vi "Logging Message Loop.vi"(8 "System Control":refnum<queue>, 10 "Data Queue":refnum<queue>, 11 "Logging":refnum<queue>) -> (0 "error out":errorcluster)   [LabVIEW 2020, in "ChromTech Next Gen Pump.lvlib" / "Logging.lvlib"]
doc: "The message loop subVI to handle messages pertaining to logging data."
uses:
  Logging.lvlib
  support/Message Queue/Message Cluster.ctl
  Instrument Manager/Instrument State.ctl
  Logging State.ctl
  Logging Configuration.ctl
  <vilib>/Utility/error.llb/Error Cluster From Error Code.vi
  <vilib>/Utility/file.llb/Write Delimited Spreadsheet (string).vi
  <vilib>/ErrorRing/Error Ring.xnode
  support/Message Queue/Message Queue.lvlib
  Instrument Manager/Instrument Manager.lvlib
panel:
  in  "error in (no error)":errorcluster
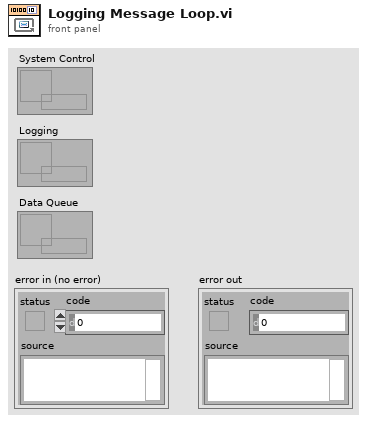
[diagram p1: front panel]
types:
  T1 = typedef "ChromTech Next Gen Pump.lvlib/Logging.lvlib/Logging Configuration.ctl" = cluster{"Log Directory Path":path, "Log File Path":path, "Log File Prefix":string, "Log File Extension":string, "File Delimiter":string, "Header Info":string[][], "Channels":string[], "Log Instrument Runs":bool}
  T2 = typedef "ChromTech Next Gen Pump.lvlib/Logging.lvlib/Logging State.ctl" = enum16{"Idle", "Logging"}
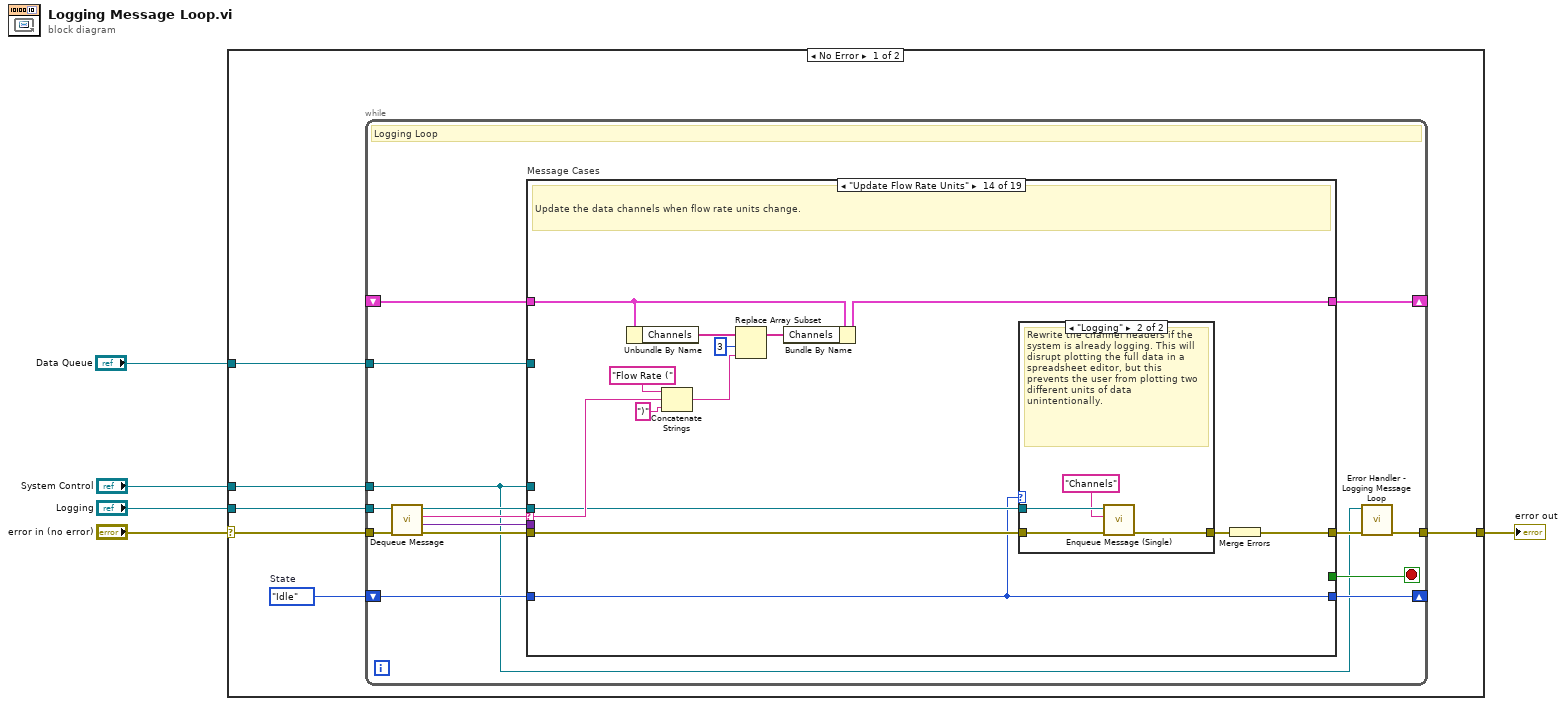
[diagram p0: block diagram]
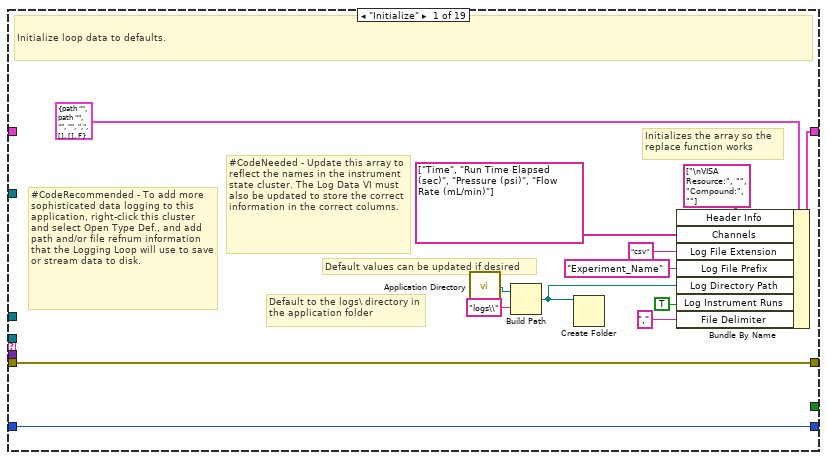
[diagram p2: hidden frame]
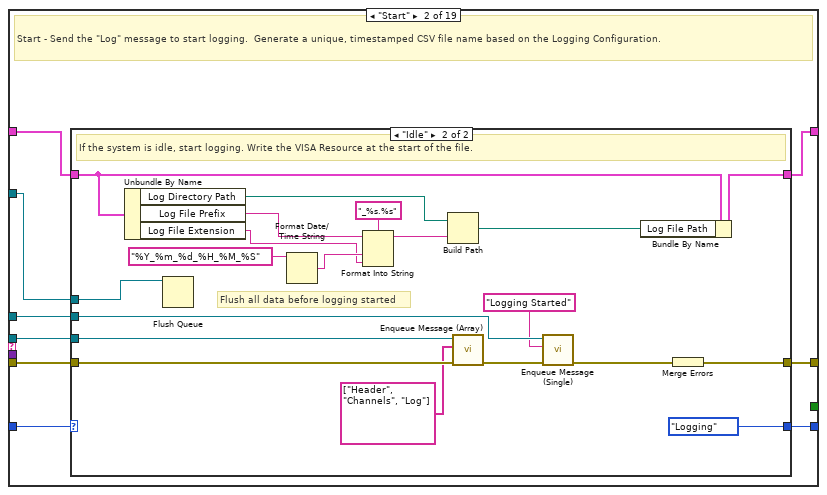
[diagram p3: hidden frame]
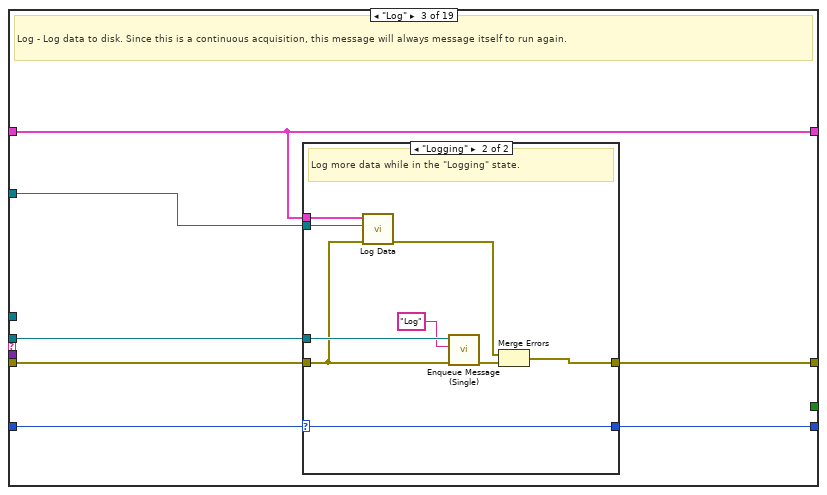
[diagram p5: hidden frame]
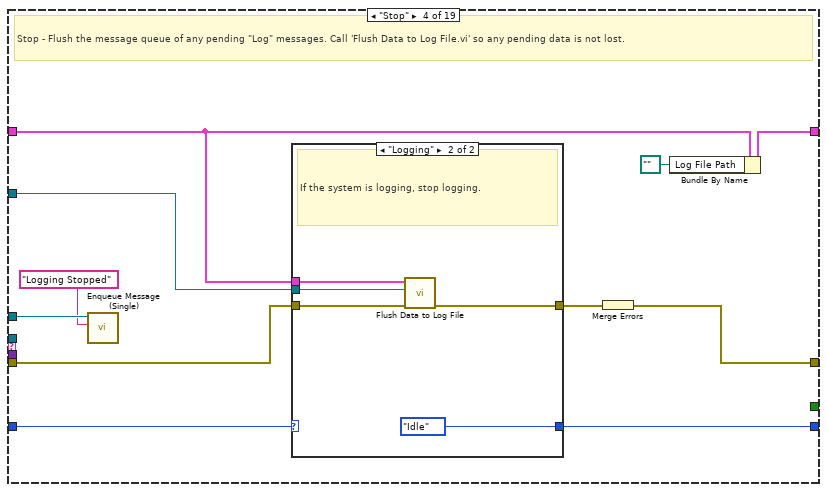
[diagram p7: hidden frame]
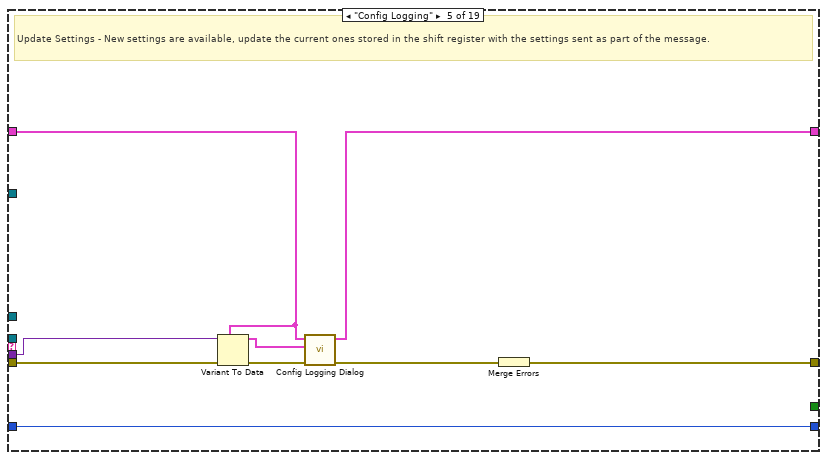
[diagram p9: hidden frame]
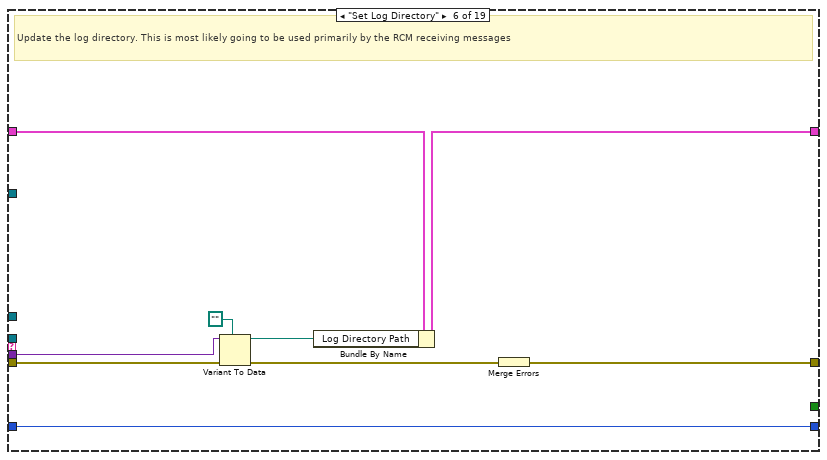
[diagram p10: hidden frame]
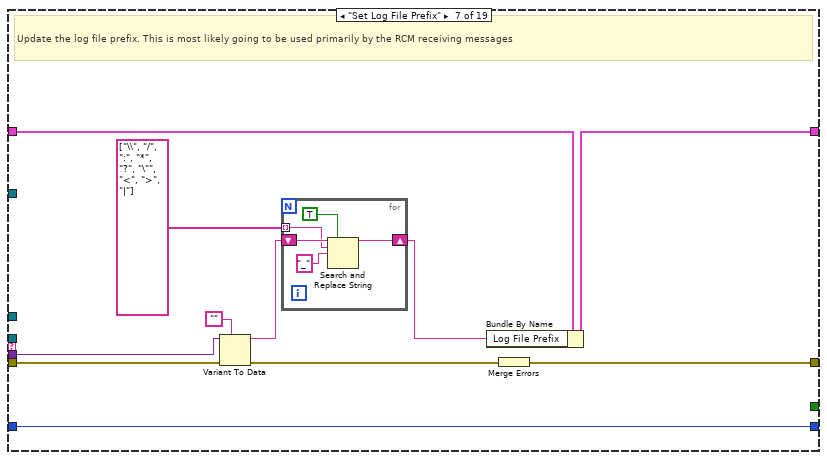
[diagram p11: hidden frame]
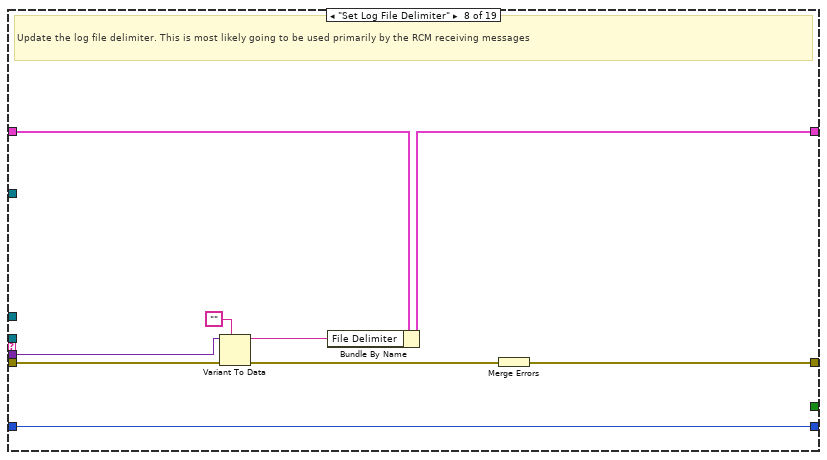
[diagram p12: hidden frame]
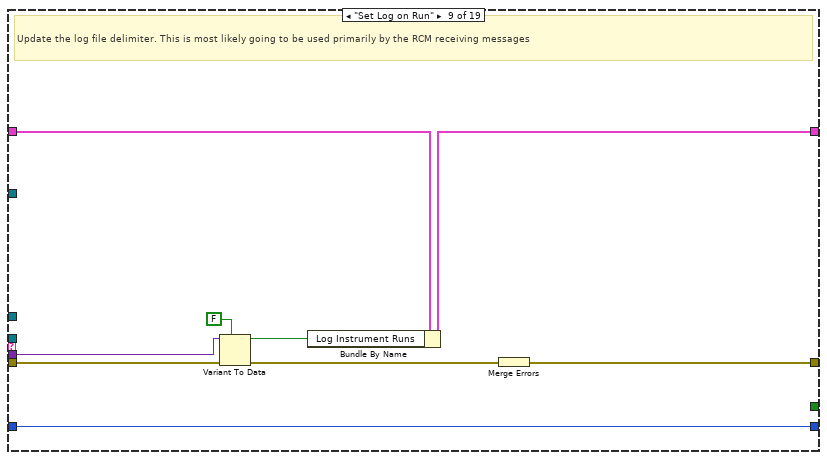
[diagram p13: hidden frame]
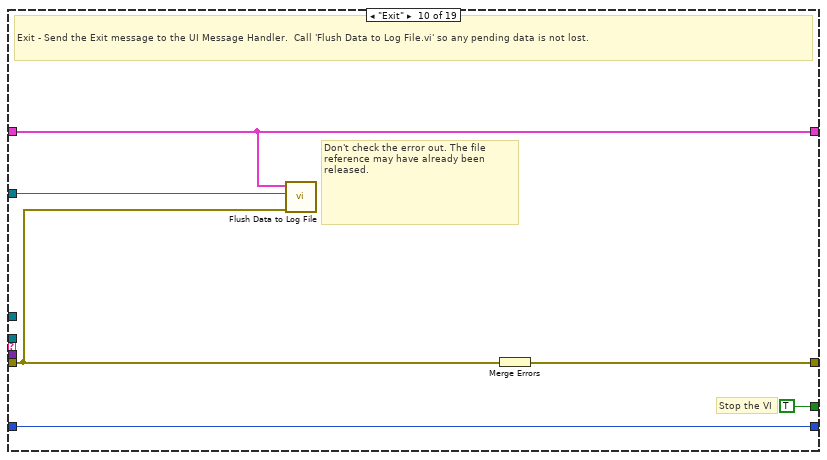
[diagram p14: hidden frame]
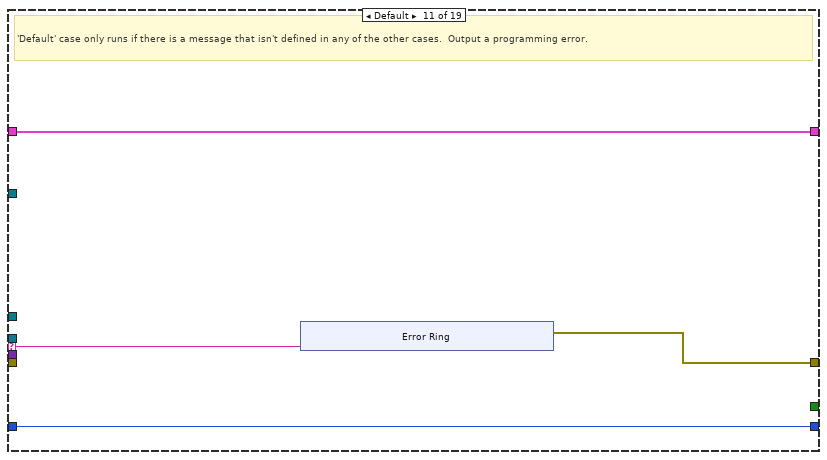
[diagram p15: hidden frame]
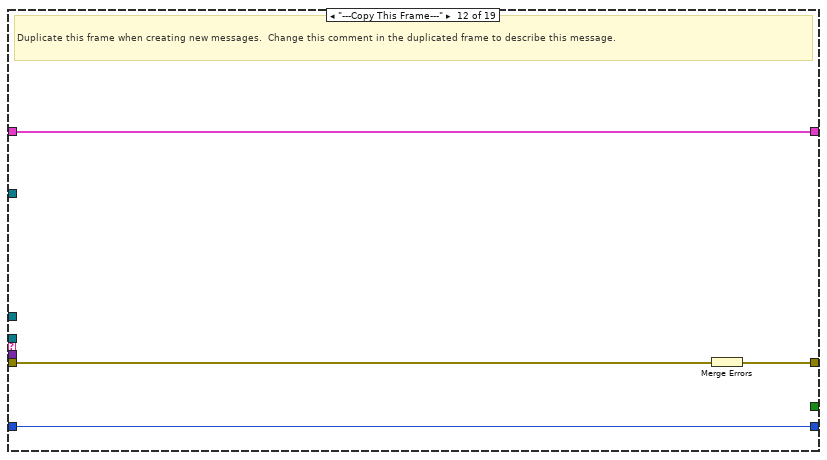
[diagram p16: hidden frame]
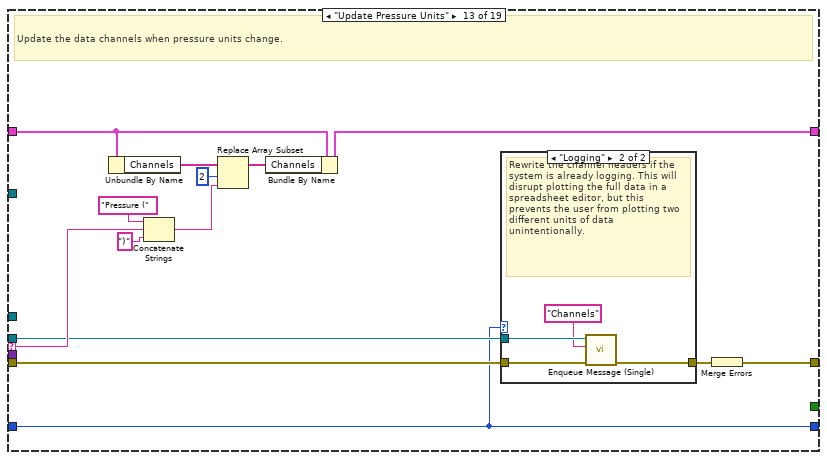
[diagram p17: hidden frame]
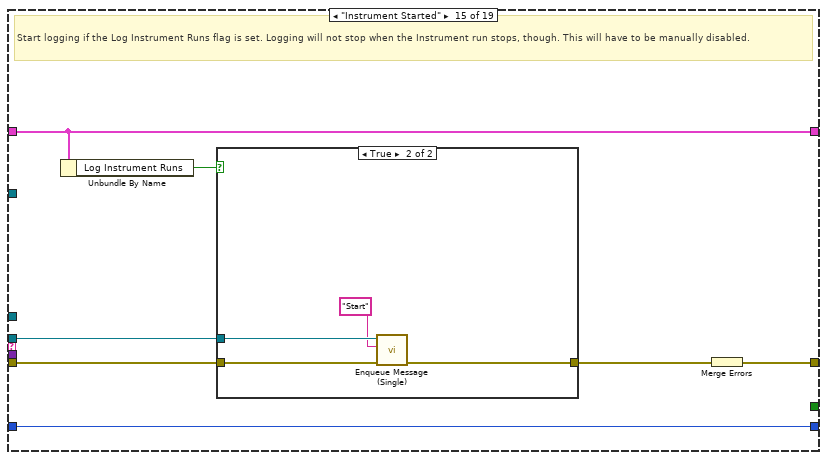
[diagram p20: hidden frame]
diagram:
  n1 = case shown="No Error" "error in (no error)" {
    selector: "error in (no error)" -> [w10 w272]
    tunnel: [w11 w272] -> w5
    tunnel: "Data Queue" -> [w9 _]
    tunnel: "System Control" -> [w7 _]
    tunnel: "Logging" -> [w6 _]
    frame No Error {
      w8 = Logging_State."Idle"  # State
      n2 = while {
        tunnel: w6 -> [w18]
        shift-right: [w25] -> _
        shift-left: _ -> [w26]
        tunnel: w7 -> [w12]
        tunnel: w9 -> [w17]
        shift-right: [w15] -> _
        shift-left: w8 -> [w16]
        tunnel: w10 -> [w23]
        tunnel: [w14] -> w11
        stop <- w24 stop-if-true
        # "Logging Loop"
        n3 = call "Dequeue Message.vi"("error in (no error)"=w23, "Message Queue"=w18) -> ("error out"=w22:errorcluster, "Message Data"=w20:variant, "Message"=w21:string, "dup Message Queue"=w19:refnum<queue>)  [unwired: 6 in]
        n4 = case "Message Cases" shown="\"Update Flow Rate Units\"" w21 {
          selector: w21 -> [_ _ _ _ _ _ _ _ _ _ w166 _ w183 w202 _ _ _ _ _]
          tunnel: w19 -> [_ w47 w77 _ _ _ _ _ _ _ _ _ w182 w201 w219 _ _ _ _]
          tunnel: w22 -> [w39 w46 w75 w95 w112 w121 w133 w146 w155 w163 _ w180 w187 w206 w221 w242 w254 w262 w269]
          tunnel: [w39 w48 w78 w100 w116 w125 w136 w150 w159 w164 w167 w178 w194 w213 w225 w241 w253 w261 w271] -> w13
          tunnel: w26 -> [_ w45 w74 w96 w109 w118 w130 w143 w152 w162 w169 w179 w185 w204 w223 w238 w250 w259 w267]
          tunnel: [w36 w44 w74 w98 w115 w117 w129 w142 w151 w162 w169 w179 w184 w203 w223 w239 w251 w259 w267] -> w25
          tunnel: [_ _ _ _ _ _ _ _ _ TRUE _ _ _ _ _ _ _ _ _] -> w24
          tunnel: w20 -> [_ _ _ _ w110 w119 w131 w144 w153 _ _ _ _ _ _ w235 w247 _ _]
          tunnel: w12 -> [_ w40 _ w91 _ _ _ _ _ _ _ _ _ _ _ _ _ _ _]
          tunnel: w17 -> [_ w41 w76 w97 _ _ _ _ _ w161 _ _ _ _ _ _ _ _ _]
          tunnel: w16 -> [w38 w43 w73 w94 w114 w124 w135 w149 w158 w160 w168 w177 w181 w200 w224 w240 w252 w260 w270]
          tunnel: [w38 w42 w72 w93 w114 w124 w135 w149 w158 w160 w168 w177 w181 w200 w224 w240 w252 w260 w270] -> w15
          frame "Initialize" {
            # "Default to the logs\\ directory in the application folder"
            # "Initializes the array so the replace function works"
            # "Default values can be updated if desired"
            # "#CodeRecommended - To add more sophisticated data logging to this application, right-click this cluster and select Open Type Def., and add path and/or file refnum information that the Logging Loop will use to save or stream data to disk."
            # "#CodeNeeded - Update this array to reflect the names in the instrument state cluster. The Log Data VI must also be updated to store the correct information in the correct columns."
            # "Initialize loop data to defaults."
            n5 = call <vilib>:"Application Directory.vi"() -> ("Application Directory"=w29:path)
            n6 = Build Path(base path=w29, name or relative path="logs\\") -> (appended path=w27:path)
            n7 = Create Folder(path (use dialog)=w27) -> ()  [unwired: 2 in, 3 out]
            n8 = Bundle By Name(cluster=T1 {"Log Directory Path"=path "", "Log File Path"=path "", "Log File Prefix"="", "Log File Extension"="", "File Delimiter"=",", "Header Info"=[], "Channels"=[], "Log Instrument Runs"=FALSE} ("Logging Configuration"), "Header Info"=string[][] [["\nVISA Resource:", ""], ["Compound:", ""]], "Channels"=string[] ["Time", "Run Time Elapsed (sec)", "Pressure (psi)", "Flow Rate (mL/min)"], "Log File Extension"="csv", "Log File Prefix"="Experiment_Name", "Log Directory Path"=w27, "Log Instrument Runs"=TRUE, "File Delimiter"=",") -> (w36:T1)
          }
          frame "Start" {
            # "Start - Send the \"Log\" message to start logging.  Generate a unique, timestamped CSV file name based on the Logging Configuration."
            n9 = case shown="\"Idle\"" w43 {
              selector: w43 -> [w50 _]
              tunnel: [w49 w63] -> w48
              tunnel: w47 -> [_ w64]
              tunnel: w46 -> [w49 w62]
              tunnel: w45 -> [w51 w65]
              tunnel: [w51 w67] -> w44
              tunnel: [w50 Logging_State."Logging" ("State")] -> w42
              tunnel: w41 -> [_ w57]
              tunnel: w40 -> [_ w53]
              frame "Logging" {
                # "The system is already logging. Ignore the \"Start\" message."
              }
              frame "Idle" {
                # "Flush all data before logging started"
                # "If the system is idle, start logging. Write the VISA Resource at the start of the file."
                n10 = Unbundle By Name(w65) -> ("Log Directory Path"=w71:path, "Log File Prefix"=w58:string, "Log File Extension"=w55:string)
                n11 = Flush Queue(queue=w57) -> ()  [unwired: 1 in, 3 out]
                n12 = Format Date/Time String(time format string (%c)="%Y_%m_%d_%H_%M_%S") -> (date/time string=w56:string)  [unwired: 2 in]
                n13 = Format Into String(format string="_%s.%s", initial string=w58, w56, w55) -> (resulting string=w69:string)  [unwired: 1 in, 1 out]
                n14 = Build Path(base path=w71, name or relative path=w69) -> (appended path=w61:path)
                n15 = call "Enqueue Message (Array).vi"("error in (no error)"=w62, "Message Array"=string[] ["Header", "Channels", "Log"], "Message Queue"=w64) -> ("error out"=w68:errorcluster)  [unwired: 7 in, 1 out]
                n16 = call "Enqueue Message (Single).vi"("error in (no error)"=w68, "Message"="Logging Started", "Message Queue"=w53) -> ("error out"=w54:errorcluster)  [unwired: 7 in, 1 out]
                n17 = Bundle By Name(cluster=w65, "Log File Path"=w61) -> (w67:T1)
                n18 = Merge Errors(w54) -> (w63:errorcluster)
              }
            }
          }
          frame "Log" {
            # "Log - Log data to disk. Since this is a continuous acquisition, this message will always message itself to run again."
            n19 = case shown="\"Logging\"" w73 {
              selector: w73 -> [w80 w83]
              tunnel: [w79 w89] -> w78
              tunnel: w77 -> [_ w87]
              tunnel: w76 -> [_ w81]
              tunnel: w75 -> [w79 w82]
              tunnel: w74 -> [_ w84]
              tunnel: [w80 w83] -> w72
              frame "Idle" {
                # "Ignore \"Log\" messages when the logging is idle."
              }
              frame "Logging" {
                # "Log more data while in the \"Logging\" state."
                n20 = call "Log Data.vi"("error in (no error)"=w82, "Data Queue"=w81, "Logging Configuration"=w84) -> ("error out"=w86:errorcluster)  [unwired: 8 in]
                n21 = call "Enqueue Message (Single).vi"("error in (no error)"=w82, "Message"="Log", "Message Queue"=w87) -> ("error out"=w88:errorcluster)  [unwired: 7 in, 1 out]
                n22 = Merge Errors(w86, w88) -> (w89:errorcluster)
              }
            }
          }
          frame "Stop" {
            # "Stop - Flush the message queue of any pending \"Log\" messages. Call 'Flush Data to Log File.vi' so any pending data is not lost."
            n23 = call "Enqueue Message (Single).vi"("Message"="Logging Stopped", "Message Queue"=w91) -> ()  [unwired: 8 in, 2 out]
            n24 = case shown="\"Logging\"" w94 {
              selector: w94 -> [w101 _]
              tunnel: [w102 w107] -> w99
              tunnel: w97 -> [_ w106]
              tunnel: w96 -> [_ w105]
              tunnel: w95 -> [w102 w104]
              tunnel: [w101 Logging_State."Idle" ("State")] -> w93
              frame "Idle" {
                # "The system is already idle. Ignore the \"Stop\" message."
              }
              frame "Logging" {
                # "If the system is logging, stop logging."
                n25 = call "Flush Data to Log File.vi"("error in (no error)"=w104, "Data Queue"=w106, "Logging Configuration"=w105) -> ("error out"=w107:errorcluster)  [unwired: 8 in]
              }
            }
            n26 = Merge Errors(w99) -> (w100:errorcluster)
            n27 = Bundle By Name(cluster=w96, "Log File Path"=path "") -> (w98:T1)
          }
          frame "Config Logging" {
            # "Update Settings - New settings are available, update the current ones stored in the shift register with the settings sent as part of the message."
            n28 = Variant To Data(error in=w112, type=w109, Variant=w110) -> (data=w108:T1, error out=w111:errorcluster)
            n29 = call "Config Logging Dialog.vi"("error in (no error)"=w111, "New Config (in)"=w108, "Current Config"=w109) -> ("error out"=w113:errorcluster, "New Config (out)"=w115:T1)  [unwired: 7 in]
            n30 = Merge Errors(w113) -> (w116:errorcluster)
          }
          frame "Set Log Directory" {
            # "Update the log directory. This is most likely going to be used primarily by the RCM receiving messages"
            n31 = Variant To Data(error in=w121, type=path "", Variant=w119) -> (data=w122:path, error out=w120:errorcluster)
            n32 = Bundle By Name(cluster=w118, "Log Directory Path"=w122) -> (w117:T1)
            n33 = Merge Errors(w120) -> (w125:errorcluster)
          }
          frame "Set Log File Prefix" {
            # "Update the log file prefix. This is most likely going to be used primarily by the RCM receiving messages"
            n34 = Variant To Data(error in=w133, type="", Variant=w131) -> (data=w127:string, error out=w132:errorcluster)
            n35 = for {
              shift-right: [w138] -> w126
              shift-left: w127 -> [w140]
              tunnel: string[] ["\\", "/", ":", "*", "?", "\"", "<", ">", "|"] -> [w139] mode=indexing
              n36 = Search and Replace String(replace all?=TRUE ("replace all? (F)"), input string=w140, search string=w139, replace string="_" ("replace string (\"\")")) -> (result string=w138:string)  [unwired: 4 in, 3 out]
            }
            n37 = Bundle By Name(cluster=w130, "Log File Prefix"=w126) -> (w129:T1)
            n38 = Merge Errors(w132) -> (w136:errorcluster)
          }
          frame "Set Log File Delimiter" {
            # "Update the log file delimiter. This is most likely going to be used primarily by the RCM receiving messages"
            n39 = Variant To Data(error in=w146, type="", Variant=w144) -> (data=w147:string, error out=w145:errorcluster)
            n40 = Bundle By Name(cluster=w143, "File Delimiter"=w147) -> (w142:T1)
            n41 = Merge Errors(w145) -> (w150:errorcluster)
          }
          frame "Set Log on Run" {
            # "Update the log file delimiter. This is most likely going to be used primarily by the RCM receiving messages"
            n42 = Variant To Data(error in=w155, type=FALSE, Variant=w153) -> (data=w156:bool, error out=w154:errorcluster)
            n43 = Bundle By Name(cluster=w152, "Log Instrument Runs"=w156) -> (w151:T1)
            n44 = Merge Errors(w154) -> (w159:errorcluster)
          }
          frame "Exit" {
            # "Don't check the error out. The file reference may have already been released."
            # "Stop the VI"
            # "Exit - Send the Exit message to the UI Message Handler.  Call 'Flush Data to Log File.vi' so any pending data is not lost."
            n45 = call "Flush Data to Log File.vi"("error in (no error)"=w163, "Data Queue"=w161, "Logging Configuration"=w162) -> ()  [unwired: 8 in, 1 out]
            n46 = Merge Errors(w163) -> (w164:errorcluster)
          }
          frame Default {
            # "'Default' case only runs if there is a message that isn't defined in any of the other cases.  Output a programming error."
            n47 = xnode "Error Ring"("parameter 0"=w166) -> ("error out"=w167:errorcluster)
          }
          frame "---Copy This Frame---" {
            # "Duplicate this frame when creating new messages.  Change this comment in the duplicated frame to describe this message."
            n48 = Merge Errors(w180) -> (w178:errorcluster)
          }
          frame "Update Pressure Units" {
            # "Update the data channels when pressure units change."
            n49 = Unbundle By Name(w185) -> ("Channels"=w191:string[])
            n50 = Concatenate Strings("Pressure (" ("string"), w183, ")" ("string")) -> (w189:string)
            n51 = Replace Array Subset(array=w191, new element=w189, index=2) -> (w188:string[])
            n52 = Bundle By Name(cluster=w185, "Channels"=w188) -> (w184:T1)
            n53 = case shown="\"Logging\"" w181 {
              tunnel: w187 -> [w195 w199]
              tunnel: [w195 w198] -> w186
              tunnel: w182 -> [_ w197]
              frame "Idle", Default {
                # "The system is not logging. Do nothing."
              }
              frame "Logging" {
                # "Rewrite the channel headers if the system is already logging. This will disrupt plotting the full data in a spreadsheet editor, but this prevents the user from plotting two different units of data unintentionally."
                n54 = call "Enqueue Message (Single).vi"("error in (no error)"=w199, "Message"="Channels", "Message Queue"=w197) -> ("error out"=w198:errorcluster)  [unwired: 7 in, 1 out]
              }
            }
            n55 = Merge Errors(w186) -> (w194:errorcluster)
          }
          frame "Update Flow Rate Units" {
            # "Update the data channels when flow rate units change."
            n56 = Unbundle By Name(w204) -> ("Channels"=w210:string[])
            n57 = Concatenate Strings("Flow Rate (" ("string"), w202, ")" ("string")) -> (w208:string)
            n58 = Replace Array Subset(array=w210, new element=w208, index=3) -> (w207:string[])
            n59 = Bundle By Name(cluster=w204, "Channels"=w207) -> (w203:T1)
            n60 = case shown="\"Logging\"" w200 {
              tunnel: w206 -> [w214 w218]
              tunnel: [w214 w217] -> w205
              tunnel: w201 -> [_ w216]
              frame "Idle", Default {
                # "The system is not logging. Do nothing."
              }
              frame "Logging" {
                # "Rewrite the channel headers if the system is already logging. This will disrupt plotting the full data in a spreadsheet editor, but this prevents the user from plotting two different units of data unintentionally."
                n61 = call "Enqueue Message (Single).vi"("error in (no error)"=w218, "Message"="Channels", "Message Queue"=w216) -> ("error out"=w217:errorcluster)  [unwired: 7 in, 1 out]
              }
            }
            n62 = Merge Errors(w205) -> (w213:errorcluster)
          }
          frame "Instrument Started" {
            # "Start logging if the Log Instrument Runs flag is set. Logging will not stop when the Instrument run stops, though. This will have to be manually disabled."
            n63 = Unbundle By Name(w223) -> ("Log Instrument Runs"=w222:bool)
            n64 = case shown="True" w222 {
              tunnel: w221 -> [w226 w230]
              tunnel: [w226 w229] -> w220
              tunnel: w219 -> [_ w228]
              frame False {
              }
              frame True {
                n65 = call "Enqueue Message (Single).vi"("error in (no error)"=w230, "Message"="Start", "Message Queue"=w228) -> ("error out"=w229:errorcluster)  [unwired: 7 in, 1 out]
              }
            }
            n66 = Merge Errors(w220) -> (w225:errorcluster)
          }
          frame "Valid VISA Resource" {
            # "Store the valid VISA resource in the header information."
            n67 = Variant To Data(type=refnum<visa-resource-name> refnum ("VISA resource name"), Variant=w235) -> (data=w231:refnum<visa-resource-name>)  [unwired: 1 in, 1 out]
            n68 = Unbundle By Name(w238) -> ("Header Info"=w237:string[][])
            n69 = Replace Array Subset(array=w237, new element=w231, index (row)=0, index (col)=1) -> (w233:string[][])
            n70 = Bundle By Name(cluster=w238, "Header Info"=w233) -> (w239:T1)
            n71 = Merge Errors(w242) -> (w241:errorcluster)
          }
          frame "Set Compound" {
            # "Store the given compound in the header information."
            n72 = Variant To Data(type="", Variant=w247) -> (data=w244:string)  [unwired: 1 in, 1 out]
            n73 = Unbundle By Name(w250) -> ("Header Info"=w249:string[][])
            n74 = Replace Array Subset(array=w249, new element=w244, index (row)=1, index (col)=1) -> (w246:string[][])
            n75 = Bundle By Name(cluster=w250, "Header Info"=w246) -> (w251:T1)
            n76 = Merge Errors(w254) -> (w253:errorcluster)
          }
          frame "Header" {
            # "Adds header information to the file. Call this before Channels or Log."
            n77 = Unbundle By Name(w259) -> ("Log File Path"=w256:path, "Header Info"=w257:string[][], "File Delimiter"=w255:string)
            n78 = call-poly <vilib>:"Write Delimited Spreadsheet.vi"("file path (dialog if empty)"=w256, "2D data"=w257, "error in (no error)"=w262, "delimiter (\\t)"=w255) -> ("error out"=w258:errorcluster)  [unwired: 10 in, 1 out]
            n79 = Merge Errors(w258) -> (w261:errorcluster)
          }
          frame "Channels" {
            # "Adds column headers to the file. Call this before Log but after Header."
            n80 = Unbundle By Name(w267) -> ("Log File Path"=w266:path, "Channels"=w264:string[], "File Delimiter"=w263:string)
            n81 = call-poly <vilib>:"Write Delimited Spreadsheet.vi"("file path (dialog if empty)"=w266, "1D data"=w264, "append to file? (new file:F)"=TRUE, "error in (no error)"=w269, "delimiter (\\t)"=w263) -> ("error out"=w268:errorcluster)  [unwired: 9 in, 1 out]
            n82 = Merge Errors(w268) -> (w271:errorcluster)
          }
        }
        n83 = call "Error Handler - Logging Message Loop.vi"("error in (no error)"=w13, "Message Queue"=w12) -> ("dup error in"=w14:errorcluster)  [unwired: 8 in, 1 out]
      }
    }
    frame Error {
    }
  }
  "error out" <- w5
